vi "Generate Trace for Message.vi"(9 "Message Name":string, 10 "Receiver Enqueuer":refnum<class "Message Enqueuer.lvclass">) -> ()   [LabVIEW 2020, in "Actor Framework.lvlib"]
doc: "Generates a DETT User Generated Trace for a message object being sent."
uses:
  Actor Framework.lvlib
  Message Enqueuer/Message Enqueuer.lvclass
  Support/Registration Mode.ctl
  Support/TDM Registration Mode.ctl
  Support/Localized Strings.vi
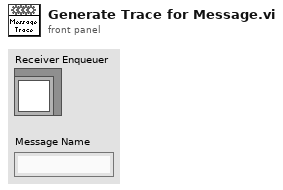
[diagram p1: front panel]
types:
  T1 = typedef "Actor Framework.lvlib/Registration Mode.ctl" = enum16{"Register Actor", "Get ID", "Get Enqueuer", "Deregister Actor", "Get Update Event", "Get All Actors"}
  T2 = typedef "Actor Framework.lvlib/TDM Registration Mode.ctl" = enum16{"Register TDM", "Get ID", "Get Notifier", "Deregister TDM"}
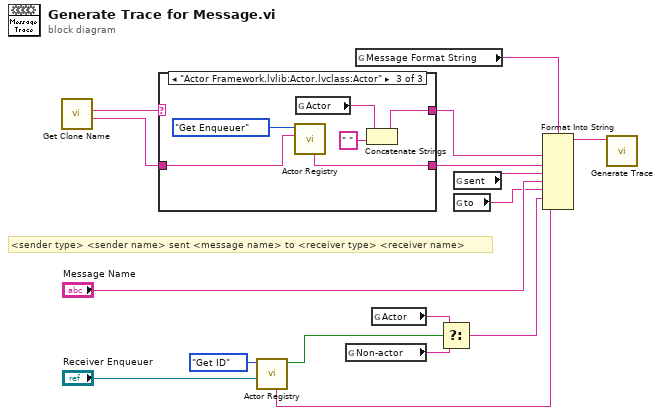
[diagram p0: block diagram]
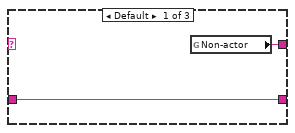
[diagram p2: hidden frame]
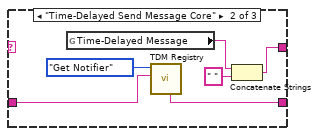
[diagram p3: hidden frame]
diagram:
  # "<sender type> <sender name> sent <message name> to <receiver type> <receiver name>"
  n1 = call "Get Clone Name.vi"() -> ("Clone ID"=w7:string, "Clone Type"=w8:string)  [unwired: 10 in]
  n2 = case shown="\"Actor Framework.lvlib:Actor.lvclass:Actor\"" w8 {
    tunnel: [w18 w24 w26] -> w14
    tunnel: w7 -> [w17 w19 w29]
    tunnel: [w17 w20 w25] -> w9
    frame Default {
      n3 = global read "Localized Strings.vi" "Non-actor"() -> (w18:string)
    }
    frame "Time-Delayed Send Message Core" {
      n4 = global read "Localized Strings.vi" "Time-Delayed Message"() -> (w22:string)
      n5 = call "TDM Registry.vi"("TDM ID"=w19, "Action"=TDM_Registration_Mode."Get Notifier") -> ("TDM Alias Out"=w20:string)  [unwired: 5 in, 4 out]
      n6 = Concatenate Strings(w22, " " ("string")) -> (w24:string)
    }
    frame "Actor Framework.lvlib:Actor.lvclass:Actor" {
      n7 = call "Actor Registry.vi"("Actor ID"=w29, "Action"=Registration_Mode."Get Enqueuer") -> ("Actor Alias out"=w25:string)  [unwired: 5 in, 4 out]
      n8 = global read "Localized Strings.vi" "Actor"() -> (w27:string)
      n9 = Concatenate Strings(w27, " " ("string")) -> (w26:string)
    }
  }
  n10 = call "Actor Registry.vi"("Actor Enqueuer"="Receiver Enqueuer", "Action"=Registration_Mode."Get ID") -> ("Found"=w13:bool, "Actor Alias out"=w11:string)  [unwired: 5 in, 3 out]
  n11 = global read "Localized Strings.vi" "Non-actor"() -> (w5:string)
  n12 = global read "Localized Strings.vi" "Message Format String"() -> (w4:string)
  n13 = global read "Localized Strings.vi" "Actor"() -> (w6:string)
  n14 = Select(t=w6, s=w13, f=w5) -> (s? t:f=w12:string)
  n15 = global read "Localized Strings.vi" "sent"() -> (w3:string)
  n16 = global read "Localized Strings.vi" "to"() -> (w2:string)
  n17 = Format Into String(format string=w4, w14, w9, w3, "Message Name", w2, w12, w11) -> (resulting string=w1:string)  [unwired: 2 in, 1 out]
  n18 = call "Generate Trace.vi"("String"=w1) -> ()  [unwired: 11 in]
